vi "Read.vi"(8 "error in":errorcluster, 11 "ChillerNew.lvclass":refnum<class "ChillerNew.lvclass">) -> (0 "error out":errorcluster, 2 "Data out":T1, 3 "output cluster":refnum<class "ChillerNew.lvclass">)   [LabVIEW 2023, in "ChillerNew.lvclass"]
uses:
  ChillerNew.lvclass
  ChillerNew.lvclass/ChillerNew.ctl
  9c8d422d-920d-4f62-ba29-e6a76558d5ae.vi
  9c8d422d-920d-4f62-ba29-e6a76558d5ae.vi/c28b0ead-42ad-4072-80a2-aca7f2bd7ce3.vi
  9c8d422d-920d-4f62-ba29-e6a76558d5ae.vi/219d0231-d98b-4193-b5cc-84f90e3c9091.vi
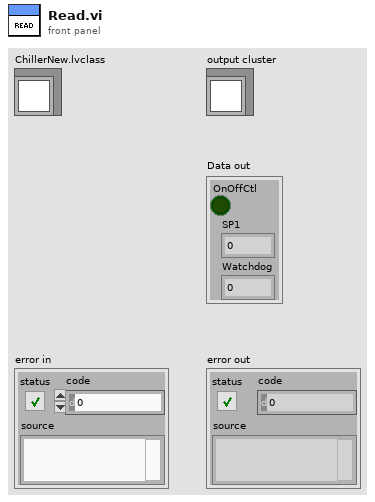
[diagram p1: front panel]
types:
  T1 = cluster{"OnOffCtl":bool, "SP1":dbl, "Watchdog":i32}
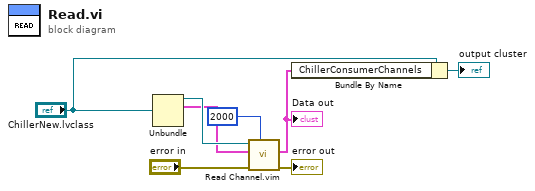
[diagram p0: block diagram]
diagram:
  n1 = Unbundle("ChillerNew.lvclass") -> (w2:refnum<k21>, w1:T1)  [unwired: 2 out]
  n2 = call "Read Channel.vim"("Timeout (ms)"=2000, "error in"="error in", "Data in"=w1, "ADAS HIL Channel in"=w2) -> ("error out"=→"error out":errorcluster, "Data out"=w5:T1)  [unwired: 4 in, 2 out]
  "Data out" <- w5
  n3 = Bundle By Name(cluster="ChillerNew.lvclass", "ChillerConsumerChannels"=w5) -> (→"output cluster":refnum<class "ChillerNew.lvclass">)
